vi "Authorization License File Creation GUI.vi"() -> ()   [LabVIEW 2011]
uses:
  OASIS/OASIS.LIB/AUTHORIZE/OBJLIB/PRIVATE/CORE Options.ctt
  SPARTAN/license/Authorization Data.ctl
panel:
  in  "Customer":string
  in  "Expiration Date":timestamp
  in  "Exit":bool
  in  "Generate":bool
  out "Product Features":enum32{"Spartan", "Oasis", "PIM"}(tab)
  in  "Seats":i32=1
  in  "Spartan Features":T1={"Attenuator"=FALSE, "DC Attenuation"=FALSE, "PIM"=FALSE, "Power Accuracy"=FALSE, "Power Output"=FALSE, "Prompt"=TRUE, "Prompted Inputs"=TRUE, "S Parameter"=FALSE, "Switch"=FALSE} caption="Features"
  in  "USB Key?":bool
  in  "Oasis Features":T2={"Core"=TRUE, "Emitter Manager"=TRUE, "Interference Manager"=TRUE, "FCC Database"=TRUE, "Scheduler"=TRUE, "Drive Test"=TRUE, "TBD Option 3"=FALSE, "TBD Option 4"=FALSE, "US Map"=TRUE, "Europe Map"=FALSE, "China Map"=FALSE, "Africa Map"=FALSE, "North-South America Map"=FALSE, "10 Drivers"=FALSE, "25 Drivers"=FALSE, "50 Drivers"=FALSE, "Advantest"=FALSE, "Agilent"=TRUE, "Future"=FALSE, "Anritsu"=TRUE, "Future"=FALSE, "Future"=FALSE, "Rohde & Schwarz"=TRUE, "Spectrum Analyzer Simulator"=TRUE, "Willtek 9100"=FALSE, "NetTek"=FALSE, "NI 5660"=FALSE, "Future"=FALSE, "ICOM"=FALSE, "Future"=FALSE, "Future"=FALSE, "Future"=FALSE} caption="Features"
  in  "Product":enum32{"Spartan", "Oasis", "PIM"}(radio)
  in  "Product Serial Number":string
  in  "Hardware ID (machine site code)":string
  in  "License File Path (Prompt if blank)":path
  # "* Required"
  # "* Required"
  # "* Required"
  # "If USB key is selected, the license file\npath must be the USB key drive."
  # "Authorization not Implemented."
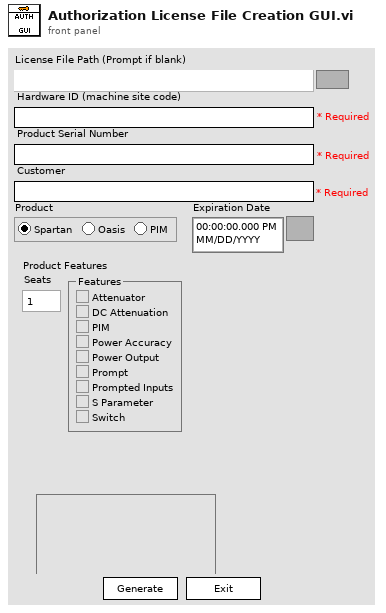
[diagram p1: front panel]
types:
  T1 = cluster{"Attenuator":bool, "DC Attenuation":bool, "PIM":bool, "Power Accuracy":bool, "Power Output":bool, "Prompt":bool, "Prompted Inputs":bool, "S Parameter":bool, "Switch":bool}
  T2 = cluster{"Core":bool, "Emitter Manager":bool, "Interference Manager":bool, "FCC Database":bool, "Scheduler":bool, "Drive Test":bool, "TBD Option 3":bool, "TBD Option 4":bool, "US Map":bool, "Europe Map":bool, "China Map":bool, "Africa Map":bool, "North-South America Map":bool, "10 Drivers":bool, "25 Drivers":bool, "50 Drivers":bool, "Advantest":bool, "Agilent":bool, "Future":bool, "Anritsu":bool, "Future":bool, "Future":bool, "Rohde & Schwarz":bool, "Spectrum Analyzer Simulator":bool, "Willtek 9100":bool, "NetTek":bool, "NI 5660":bool, "Future":bool, "ICOM":bool, "Future":bool, "Future":bool, "Future":bool}
  T3 = typedef "CORE Options.ctt" = cluster{"CORE":bool, "Emitter Manager":bool, "Interference Manager":bool, "FCC Database":bool, "Scheduler":bool, "Drive Test":bool, "TBD Option 3":bool, "TBD Option 4":bool, "US Map":bool, "Europe Map":bool, "China Map":bool, "Africa":bool, "North-South America":bool, "10 Drivers":bool, "25 Drivers":bool, "50 Drivers":bool, "Advantest":bool, "Agilent":bool, "Future":bool, "Anritsu":bool, "Future":bool, "Future":bool, "Rohde & Schwarz":bool, "Spectrum Analyzer Simulator":bool, "Willtek 9100":bool, "NetTek":bool, "NI 5660":bool, "Future":bool, "ICOM":bool, "Future":bool, "Future":bool, "Future":bool}
  T4 = enum16{"open", "replace", "create", "open or create", "replace or create", "replace or create with confirmation"}
  T5 = enum8{"Enabled", "Disabled", "Disabled and Grayed Out"}
  T6 = typedef "LVDateTimeRec.ctl" = cluster{"fractional second":dbl, "second":i32, "minute":i32, "hour":i32, "day of month":i32, "month":i32, "year":i32, "day of week":i32, "day of year":i32, "DST":i32}
  T7 = typedef "Authorization Data.ctl" = cluster{"Valid":bool, "Seats":i32, "Expire Time":timestamp, "Last Access Time":timestamp, "Product ID":string, "Hardware ID":string, "Spartan Serial Number":string, "Feature":cluster{"#attributes":cluster{"Name":string, "Value":string}}[]}
  T8 = cluster{"#attributes":cluster{"Name":string, "Value":string}}
  T9 = enum32{"invalid app kind", "Development System", "Run Time System", "Student Edition", "Embedded LabVIEW", "Evaluation", "Custom"}
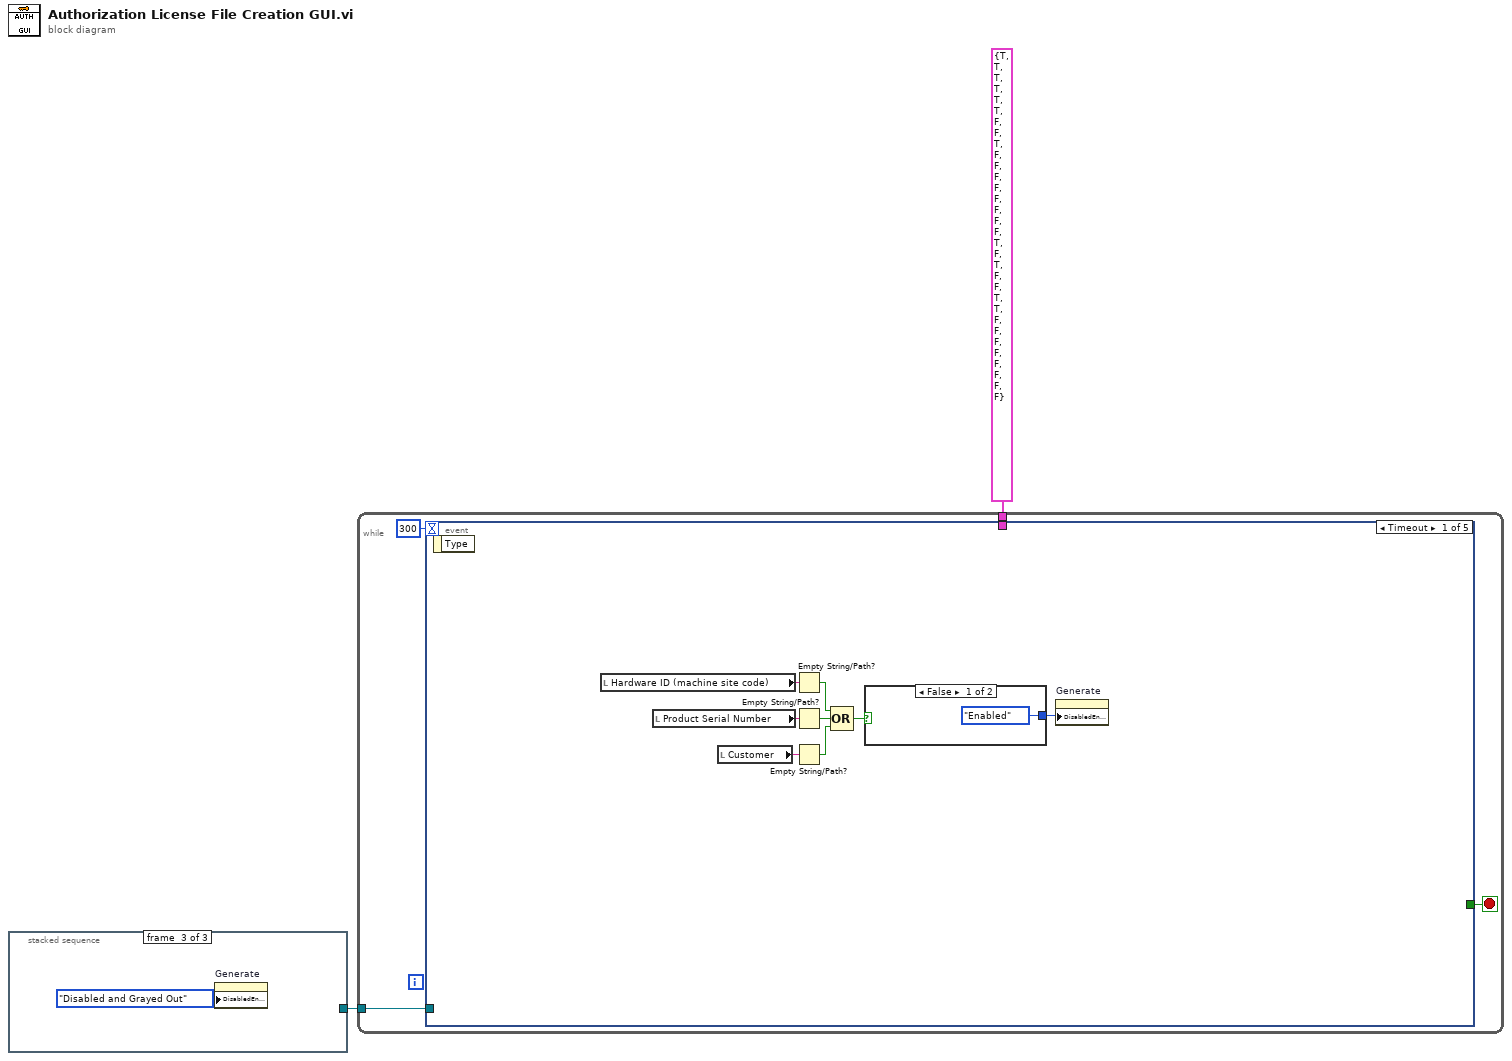
[diagram p0: block diagram]
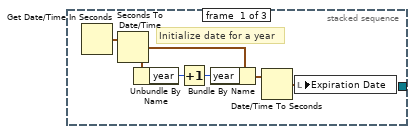
[diagram p2: hidden frame]
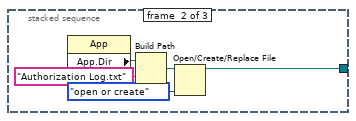
[diagram p3: hidden frame]
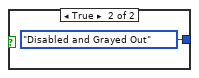
[diagram p4: hidden frame]
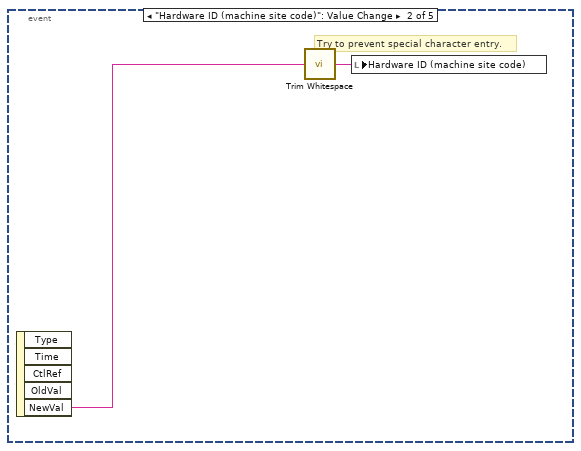
[diagram p5: hidden frame]
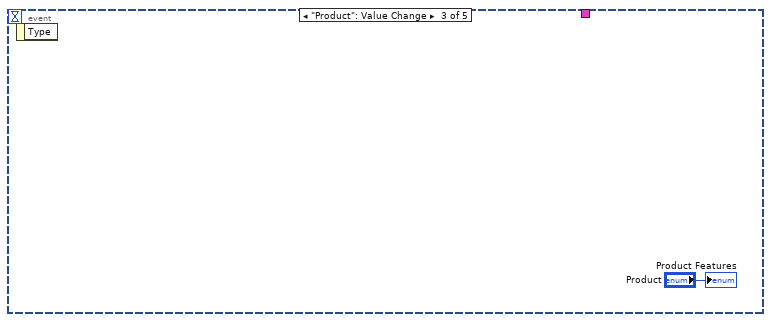
[diagram p6: hidden frame]
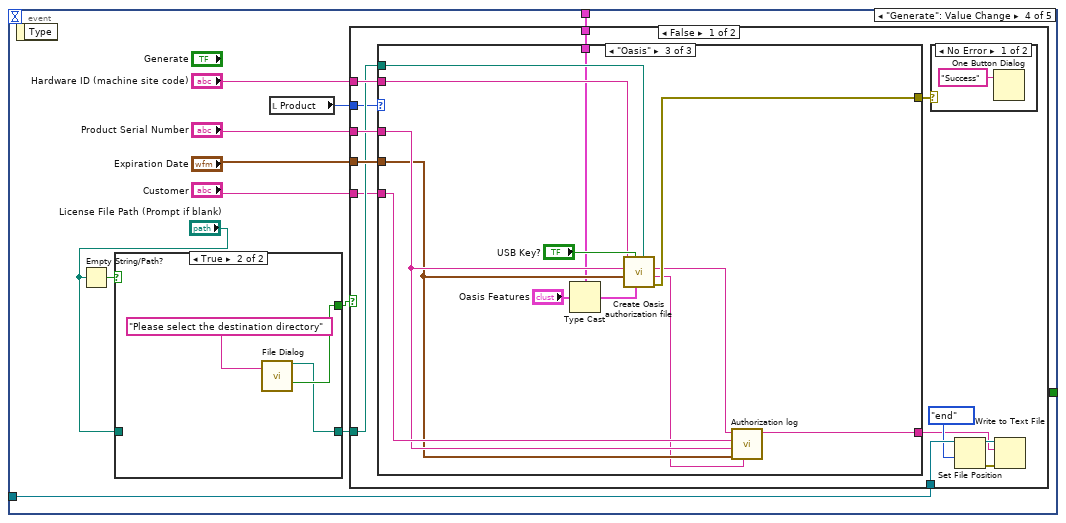
[diagram p7: hidden frame]
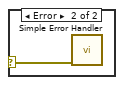
[diagram p9: hidden frame]
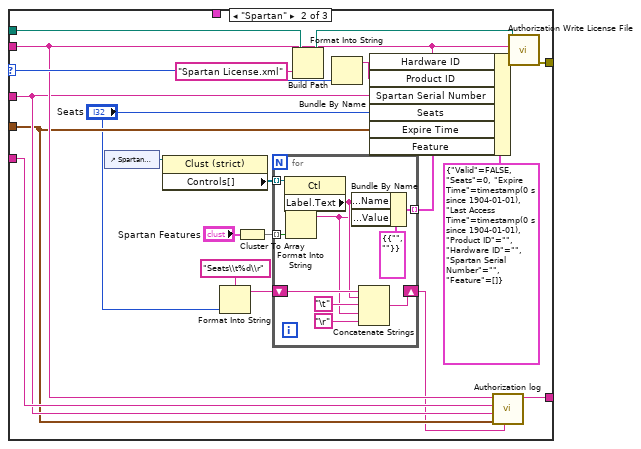
[diagram p11: hidden frame]
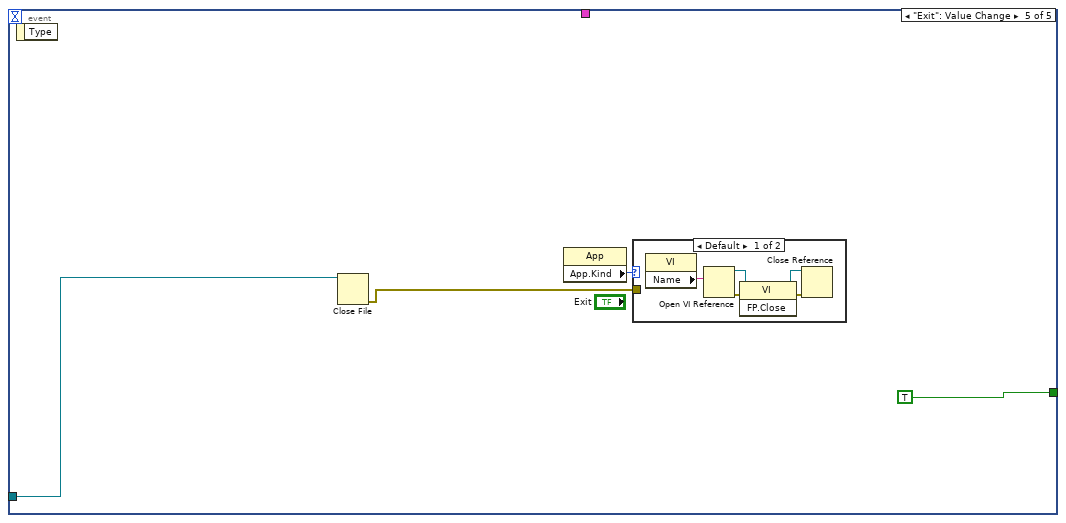
[diagram p13: hidden frame]
diagram:
  n1 = stacked-sequence {
    tunnel: [_ w9 _] -> w2
    frame #0 {
      # "Initialize date for a year"
      n2 = Get Date/Time In Seconds() -> (seconds since 1Jan1904=w8:timestamp)
      n3 = Seconds To Date/Time(time stamp (now)=w8) -> (date time rec=w6:T6)  [unwired: 1 in]
      n4 = Unbundle By Name(w6) -> ("year"=w5:i32)
      n5 = Increment(x=w5) -> (x+1=w4:i32)
      n6 = Bundle By Name(cluster=w6, "year"=w4) -> (w7:T6)
      n7 = Date/Time To Seconds(2:w7) -> (0:w3:timestamp)  [unwired: 1 in]
      n8 = local write "Expiration Date"(w3) -> ()
    }
    frame #1 {
      n9 = property class="App"() -> ("App.Dir"=w13:path)  [unwired: 2 in, 2 out]
      n10 = Build Path(base path=w13, name or relative path="Authorization Log.txt") -> (appended path=w11:path)
      n11 = Open/Create/Replace File(file path (use dialog)=w11, operation (0:open)=T4."open or create") -> (refnum out=w9:refnum<file>)  [unwired: 4 in, 2 out]
    }
    frame #2 {
      n12 = property on="Generate" class="Bool"("DisabledEnum"=T5."Disabled and Grayed Out" ("Disabled")) -> ()  [unwired: 2 in, 2 out]
    }
  }
  n13 = while {
    tunnel: w2 -> [w16]
    tunnel: T3 {"CORE"=TRUE, "Emitter Manager"=TRUE, "Interference Manager"=TRUE, "FCC Database"=TRUE, "Scheduler"=TRUE, "Drive Test"=TRUE, "TBD Option 3"=FALSE, "TBD Option 4"=FALSE, "US Map"=TRUE, "Europe Map"=FALSE, "China Map"=FALSE, "Africa"=FALSE, "North-South America"=FALSE, "10 Drivers"=FALSE, "25 Drivers"=FALSE, "50 Drivers"=FALSE, "Advantest"=FALSE, "Agilent"=TRUE, "Future"=FALSE, "Anritsu"=TRUE, "Future"=FALSE, "Future"=FALSE, "Rohde & Schwarz"=TRUE, "Spectrum Analyzer Simulator"=TRUE, "Willtek 9100"=FALSE, "NetTek"=FALSE, "NI 5660"=FALSE, "Future"=FALSE, "ICOM"=FALSE, "Future"=FALSE, "Future"=FALSE, "Future"=FALSE} ("Core Options") -> [w15]
    stop <- w17 stop-if-true
    n14 = event shown="[0] Timeout" {
      selector: _ -> [_ _ _ _ _]
      dyn-events: _ -> [_ _ _ _ _]
      timeout: 300 -> [_ _ _ _ _]
      tunnel: [_ _ _ _ TRUE] -> w17
      tunnel: w16 -> [_ _ _ w38 w108]
      tunnel: w15 -> [_ _ _ w32 _]
      event Timeout {
        n15 = event-data() -> ()  [unwired: 1 in, 1 out]
        n16 = local read "Hardware ID (machine site code)"() -> (w24:string)
        n17 = local read "Product Serial Number"() -> (w25:string)
        n18 = local read "Customer"() -> (w26:string)
        n19 = Empty String/Path?(string/path=w24) -> (empty?=w23:bool)
        n20 = Empty String/Path?(string/path=w25) -> (empty?=w22:bool)
        n21 = Empty String/Path?(string/path=w26) -> (empty?=w21:bool)
        n22 = Compound Arithmetic op=OR(w23, w22, w21) -> (w20:bool)
        n23 = case shown="False" w20 {
          tunnel: [T5."Enabled" ("Disabled") T5."Disabled and Grayed Out" ("Disabled")] -> w19
          frame False {
          }
          frame True {
          }
        }
        n24 = property on="Generate" class="Bool"("DisabledEnum"=w19) -> ()  [unwired: 2 in, 2 out]
      }
      event "Hardware ID (machine site code)": Value Change {
        # "Try to prevent special character entry."
        n25 = event-data() -> ("NewVal"=w30:string)  [unwired: 1 in, 4 out]
        n26 = call <vilib>:"Trim Whitespace.vi"("string"=w30) -> ("trimmed string"=w29:string)  [unwired: 1 in]
        n27 = local write "Hardware ID (machine site code)"(w29) -> ()
      }
      event "Product": Value Change {
        n28 = event-data() -> ()  [unwired: 1 in, 1 out]
        "Product Features" <- "Product"
      }
      event "Generate": Value Change {
        n29 = event-data() -> ()  [unwired: 1 in, 1 out]
        n30 = Empty String/Path?(string/path="License File Path (Prompt if blank)") -> (empty?=w41:bool)
        n31 = case shown="True" w41 {
          tunnel: [_ w46] -> w42
          tunnel: [w43 w45] -> w40
          tunnel: "License File Path (Prompt if blank)" -> [w43 _]
          frame False {
          }
          frame True {
            n32 = call "File Dialog"("prompt"="Please select the destination directory") -> ("selected path"=w45:path, "cancelled"=w46:bool)  [unwired: 11 in, 2 out]
          }
        }
        n33 = local read "Product"() -> (w39:enum32{"Spartan", "Oasis", "PIM"})
        n34 = case shown="False" w42 {
          tunnel: "Hardware ID (machine site code)" -> [w59 _]
          tunnel: "Product Serial Number" -> [w58 _]
          tunnel: "Expiration Date" -> [w57 _]
          tunnel: w40 -> [w55 _]
          tunnel: w39 -> [w54 _]
          tunnel: w38 -> [w52 _]
          tunnel: "Customer" -> [w49 _]
          tunnel: w32 -> [w47 _]
          frame False {
            n35 = case shown="\"Oasis\"" w54 {
              selector: w54 -> [_ w75 _]
              tunnel: w55 -> [_ w72 w106]
              tunnel: w59 -> [_ w70 w102]
              tunnel: w58 -> [_ w67 w100]
              tunnel: w57 -> [_ w66 w99]
              tunnel: [_ w74 w105] -> w56
              tunnel: w49 -> [_ w68 w101]
              tunnel: [_ w69 w103] -> w48
              tunnel: w47 -> [_ _ w95]
              frame Default {
              }
              frame "Spartan" {
                n36 = control-ref of="Spartan Features"() -> (w78:refnum<vi>)
                n37 = property class="Clust (strict)"(reference=w78) -> ("Controls[]"=w77:refnum<vi>[])  [unwired: 1 in, 2 out]
                n38 = Format Into String(format string="Seats\\t%d\\r", "Seats") -> (resulting string=w65:string)  [unwired: 2 in, 1 out]
                n39 = Cluster To Array(cluster="Spartan Features") -> (array=w80:bool[])
                n40 = for {
                  tunnel: w80 -> [w92] mode=indexing
                  tunnel: [w91] -> w79 mode=indexing
                  tunnel: w77 -> [w90] mode=indexing
                  shift-right: [w89] -> w62
                  shift-left: w65 -> [w88]
                  n41 = property class="Ctl"(reference=w90) -> ("Label.Text"=w87:string)  [unwired: 1 in, 2 out]
                  n42 = Format Into String(w92) -> (resulting string=w85:string)  [unwired: 3 in, 1 out]
                  n43 = Bundle By Name(cluster=T8 {"#attributes"={"Name"="", "Value"=""}}, "#attributes.Name"=w87, "#attributes.Value"=w85) -> (w91:T8)
                  n44 = Concatenate Strings(w88, w87, "\t", w85, "\r") -> (w89:string)
                }
                n45 = Build Path(base path=w72, name or relative path="Spartan License.xml") -> (appended path=w71:path)
                n46 = Format Into String(w75) -> (resulting string=w76:string)  [unwired: 3 in, 1 out]
                n47 = Bundle By Name(cluster=T7 {"Valid"=FALSE, "Seats"=0, "Expire Time"=timestamp(0 s since 1904-01-01), "Last Access Time"=timestamp(0 s since 1904-01-01), "Product ID"="", "Hardware ID"="", "Spartan Serial Number"="", "Feature"=[]} ("Authorization"), "Hardware ID"=w70, "Product ID"=w76, "Spartan Serial Number"=w67, "Seats"="Seats", "Expire Time"=w66, "Feature"=w79) -> (w82:T7)
                n48 = call "Authorization log.vi"("EXTRA"=w62, "EXPIRE"=w66, "SN"=w67, "CUSTOMER"=w68, "hw ID"=w70) -> ("concatenated string"=w69:string)  [unwired: 6 in]
                n49 = call "Authorization Write License File.vi"("Authorization"=w82, "Hardware ID"=w70, "Spartan License File Path"=w71) -> ("error out"=w74:errorcluster)  [unwired: 8 in]
              }
              frame "Oasis" {
                n50 = Type Cast(type=w95, x="Oasis Features") -> (*(type *) &x=w96:T3)
                n51 = call "Create Oasis authorization file.vi"("selected path"=w106, "CORE Options"=w96, "USE USB  KEY?"="USB Key?", "Expire Date"=w99, "oasis authorization key"=w100, "user machine site code"=w102) -> ("error out"=w105:errorcluster, "Log String"=w98:string, "HW ID"=w94:string)  [unwired: 3 in]
                n52 = call "Authorization log.vi"("EXTRA"=w98, "EXPIRE"=w99, "SN"=w100, "CUSTOMER"=w101, "hw ID"=w94) -> ("concatenated string"=w103:string)  [unwired: 6 in]
              }
            }
            n53 = case shown="No Error" w56 {
              selector: w56 -> [_ w61]
              frame No Error {
                n54 = One Button Dialog(message="Success") -> ()  [unwired: 1 in, 1 out]
              }
              frame Error {
                n55 = call <vilib>:"Simple Error Handler.vi"("error in (no error)"=w61) -> ()  [unwired: 4 in, 5 out]
              }
            }
            n56 = Set File Position(refnum=w52, from (0:start)=enum16{"start", "end", "current"}."end") -> (refnum out=w51:refnum<file>, error out=w53:errorcluster)  [unwired: 2 in]
            n57 = Write to Text File(file (use dialog)=w51, text=w48, error in=w53) -> ()  [unwired: 1 in, 3 out]
          }
          frame True {
          }
        }
      }
      event "Exit": Value Change {
        n58 = event-data() -> ()  [unwired: 1 in, 1 out]
        n59 = Close File(refnum=w108) -> (error out=w107:errorcluster)  [unwired: 1 in, 1 out]
        n60 = property class="App"() -> ("App.Kind"=w110:T9)  [unwired: 2 in, 2 out]
        n61 = case shown="Default" w110 {
          tunnel: w107 -> [_ _]
          frame Default {
            n62 = property class="VI"() -> ("Name"=w111:string)  [unwired: 2 in, 2 out]
            n63 = Open VI Reference(vi path=w111) -> (vi reference=w115:refnum<vi>, error out=w114:errorcluster)  [unwired: 5 in]
            n64 = invoke class="VI" method="FP.Close"(reference=w115, error in=w114) -> (reference out=w112:refnum<vi>, error out=w113:errorcluster)  [unwired: 1 in, 1 out]
            n65 = Close Reference(reference=w112, error in (no error)=w113) -> ()  [unwired: 1 out]
          }
          frame "Development System" {
          }
        }
      }
    }
  }
